vi "KH7008 Get Channel.vi"(8 "error in (no error)":errorcluster, 10 "Channel":T2=enum."Channel 2", 11 "VISA Refnum in":refnum<visa-resource-name>="COM1") -> (0 "error out":errorcluster, 2 "Channel Parameters":T1, 3 "VISA Refnum out":refnum<visa-resource-name>)   [LabVIEW 2019, in "Instrument.KH7008.lvclass"]
uses:
  Instrument.KH7008.lvclass
  typedefs/Channel-Enum.ctl
  typedefs/SetAll-Cluster.ctl
  typedefs/Gain-Enum.ctl
  typedefs/Filter-Enum.ctl
  typedefs/Shunt-Enum.ctl
  typedefs/Coupling-Enum.ctl
  typedefs/Input Configuration-Enum.ctl
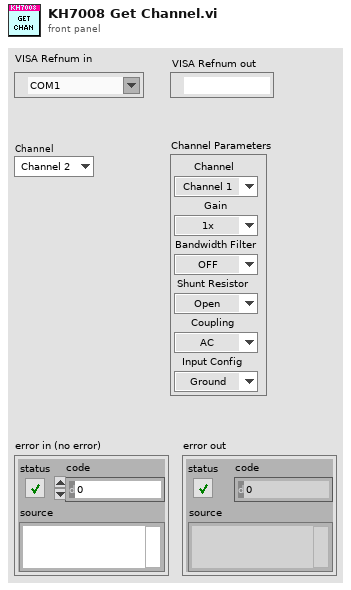
[diagram p1: front panel]
types:
  T1 = typedef "Instrument.KH7008.lvclass/SetAll-Cluster.ctl" = cluster{"Channel":T2, "Gain":T3, "Bandwidth Filter":T4, "Shunt Resistor":T5, "Coupling":T6, "Input Config":T7}
  T2 = typedef "Instrument.KH7008.lvclass/Channel-Enum.ctl" = enum16{"Channel 1", "Channel 2", "Channel 3", "Channel 4", "Channel 5", "Channel 6", "Channel 7", "Channel 8"}
  T3 = typedef "Instrument.KH7008.lvclass/Gain-Enum.ctl" = enum16{"1x", "10x", "100x", "1000x"}
  T4 = typedef "Instrument.KH7008.lvclass/Filter-Enum.ctl" = enum16{"OFF", "ON"}
  T5 = typedef "Instrument.KH7008.lvclass/Shunt-Enum.ctl" = enum16{"Open", "50 Ohms", "500 Ohms", "5k Ohms", "50k Ohms", "10M Ohm"}
  T6 = typedef "Instrument.KH7008.lvclass/Coupling-Enum.ctl" = enum16{"AC", "DC"}
  T7 = typedef "Instrument.KH7008.lvclass/Input Configuration-Enum.ctl" = enum16{"Ground", "SE+ (-gnd)", "SE- (+gnd)", "Differential"}
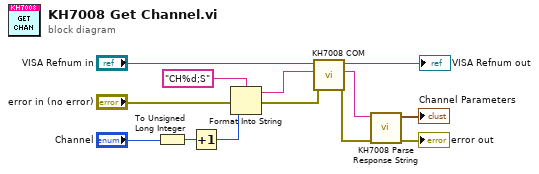
[diagram p0: block diagram]
diagram:
  n1 = To Unsigned Long Integer(number="Channel") -> (unsigned 32bit integer=w4:u32)
  n2 = Increment(x=w4) -> (x+1=w6:u32)
  n3 = Format Into String(format string="CH%d;S", error in="error in (no error)", w6) -> (resulting string=w1:string, error out=w2:errorcluster)  [unwired: 1 in]
  n4 = call "KH7008 COM.vi"("error in (no error)"=w2, "Command"=w1, "VISA Refnum in"="VISA Refnum in") -> ("error out"=w11:errorcluster, "Response"=w9:string, "VISA Refnum out"=→"VISA Refnum out":refnum<visa-resource-name>)  [unwired: 6 in]
  n5 = call "KH7008 Parse Response String.vi"("error in (no error)"=w11, "Response String"=w9) -> ("error out"=→"error out":errorcluster, "Channel Parameters"=→"Channel Parameters":T1)  [unwired: 8 in]
